vi "XL320_Configure Active Compliance.vi"(8 "error in (no error)":errorcluster, 9 "Active Compliance Settings":T1={"Clockwise Slope (9.38416 deg)"=9.384164, "Counter-Clockwise Slope (9.38416 deg)"=9.384164, "Clockwise Margin (0.293255 deg)"=0.29325512, "Counter-Clockwise Margin (0.293255 deg)"=0.29325512, "Punch (3.12805%)"=3.12805, "Max  Torque (100%)"=100.0}, 10 "Motor ID (0)":u8, 11 "VISA resource name":refnum<visa-resource-name>) -> (0 "error out":errorcluster, 3 "VISA resource name out":refnum<visa-resource-name>)   [LabVIEW 2017, in "Dynamixel XL320.lvlib"]
doc: "Adjusts the active compliance of the motor. See the motor's user manual for more details."
uses:
  <instrlib>/Dynamixel XL320 (Drivers instrument)/Dynamixel XL320.lvlib
  <instrlib>/Dynamixel XL320 (Drivers instrument)/Public/Configure/XL320_Active Compliance Settings.ctl
  <instrlib>/Dynamixel XL320 (Drivers instrument)/Public/Configure/XL320_Select_Action.ctl
panel:
  # "Ghislain REMY, IUT de Cachan, 2015 December 2015"
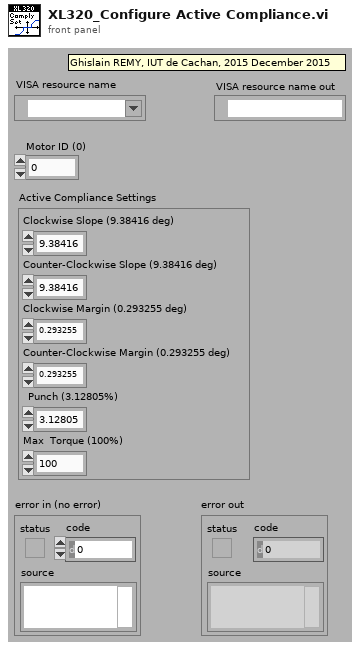
[diagram p1: front panel]
types:
  T1 = typedef "Dynamixel XL320.lvlib/XL320_Active Compliance Settings.ctl" = cluster{"Clockwise Slope (9.38416 deg)":sgl, "Counter-Clockwise Slope (9.38416 deg)":sgl, "Clockwise Margin (0.293255 deg)":sgl, "Counter-Clockwise Margin (0.293255 deg)":sgl, "Punch (3.12805%)":sgl, "Max  Torque (100%)":sgl}
  T2 = typedef "Dynamixel XL320.lvlib/XL320_Select_Action.ctl" = u8
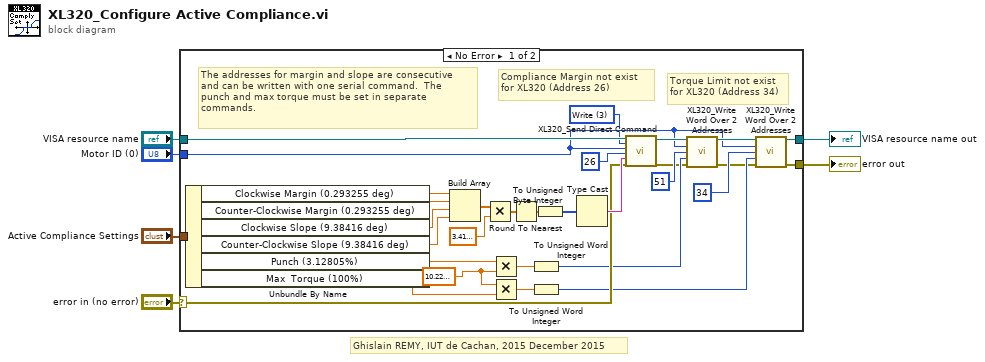
[diagram p0: block diagram]
diagram:
  # "Ghislain REMY, IUT de Cachan, 2015 December 2015"
  n1 = case shown="No Error" "error in (no error)" {
    selector: "error in (no error)" -> [w19 w39]
    tunnel: "VISA resource name" -> [w22 w38]
    tunnel: "Motor ID (0)" -> [w12 _]
    tunnel: "Active Compliance Settings" -> [w37 _]
    tunnel: [w8 w39] -> w3
    tunnel: [w13 w38] -> w2
    frame No Error {
      w7 = T2 3 items=["Ping"=1, "Read"=2, "Write"=3, "Registered Write"=4, "Action"=5, "Reset"=6, "Reboot"=8, "Status"=85, "Sync Read"=130, "Sync Write"=131, "Bulk Read"=146, "Bulk Write"=147] ("Select Action")
      w25 = sgl 10.23 ("y")
      # "Compliance Margin not exist\nfor XL320 (Address 26)"
      # "Torque Limit not exist\nfor XL320 (Address 34)"
      # "The addresses for margin and slope are consecutive \nand can be written with one serial command.  The\npunch and max torque must be set in separate\ncommands."
      n2 = Unbundle By Name(w37) -> ("Clockwise Margin (0.293255 deg)"=w36:sgl, "Counter-Clockwise Margin (0.293255 deg)"=w35:sgl, "Clockwise Slope (9.38416 deg)"=w34:sgl, "Counter-Clockwise Slope (9.38416 deg)"=w33:sgl, "Punch (3.12805%)"=w27:sgl, "Max  Torque (100%)"=w26:sgl)
      n3 = Build Array(w36, w35, w34, w33) -> (w32:sgl[])
      n4 = Multiply(x=w32, y=sgl 3.41) -> (x*y=w30:sgl[])
      n5 = Multiply(x=w27, y=w25) -> (x*y=w24:sgl)
      n6 = Multiply(x=w25, y=w26) -> (x*y=w23:sgl)
      n7 = Round To Nearest(number=w30) -> (nearest integer value=w29:sgl[])
      n8 = To Unsigned Word Integer(number=w24) -> (unsigned 16bit integer=w16:u16)
      n9 = To Unsigned Word Integer(number=w23) -> (unsigned 16bit integer=w10:u16)
      n10 = To Unsigned Byte Integer(number=w29) -> (unsigned 8bit integer=w28:u8[])
      n11 = Type Cast(x=w28) -> (*(type *) &x=w20:string)  [unwired: 1 in]
      n12 = call <instrlib>:"XL320_Send Direct Command.vi"("VISA resource name"=w22, "Select Action"=w7, "Motor ID (0)"=w12, "Address"=u16 26, "Parameters"=w20, "Error in (no error)"=w19) -> ("VISA resource name out"=w18:refnum<visa-resource-name>, "Error out"=w15:errorcluster)  [unwired: 11 in, 1 out]
      n13 = call <instrlib>:"XL320_Write Word Over 2 Addresses.vi"("VISA resource name"=w18, "Motor ID (0)"=w12, "Address number (0)"=u16 51, "Parameter (0)"=w16, "error in (no error)"=w15) -> ("VISA resource name out"=w14:refnum<visa-resource-name>, "error out"=w9:errorcluster)  [unwired: 9 in]
      n14 = call <instrlib>:"XL320_Write Word Over 2 Addresses.vi"("VISA resource name"=w14, "Motor ID (0)"=w12, "Address number (0)"=u16 34 ("Address"), "Parameter (0)"=w10, "error in (no error)"=w9) -> ("VISA resource name out"=w13:refnum<visa-resource-name>, "error out"=w8:errorcluster)  [unwired: 9 in]
    }
    frame Error {
    }
  }
  "VISA resource name out" <- w2
  "error out" <- w3
